vi "Capture_Python_Error.vi"(8 "error in (no error)":errorcluster, 11 "Error Message (start with ERROR)":string) -> (0 "error out":errorcluster)   [LabVIEW 2023]
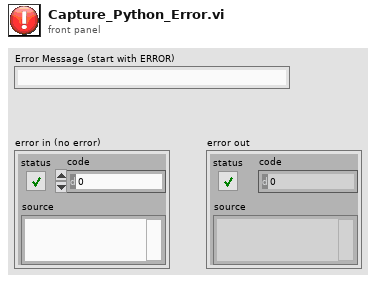
[diagram p1: front panel]
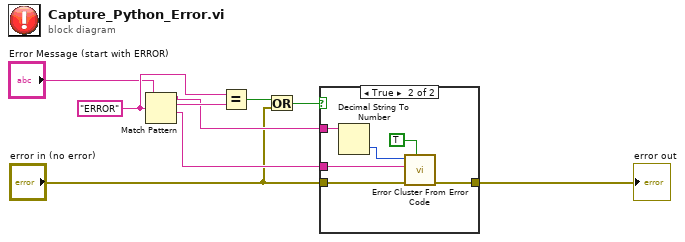
[diagram p0: block diagram]
diagram:
  w9 = "ERROR" ("regular expression")
  n1 = Match Pattern(string="Error Message (start with ERROR)", regular expression=w9) -> (before substring=w4:string, match substring=w8:string, after substring=w5:string)  [unwired: 1 in, 1 out]
  n2 = Equal?(x=w9, y=w8) -> (x = y?=w2:bool)
  n3 = Or(x=w2, y="error in (no error)") -> (x .or. y?=w1:bool)
  n4 = case shown="True" w1 {
    tunnel: "error in (no error)" -> [w10 w16]
    tunnel: [w10 w15] -> w6
    tunnel: w5 -> [_ w13]
    tunnel: w4 -> [_ w12]
    frame False {
    }
    frame True {
      n5 = Decimal String To Number(string=w12) -> (number=w11:i32)  [unwired: 2 in, 1 out]
      n6 = call <vilib>:"Error Cluster From Error Code.vi"("show call chain? (False)"=TRUE, "error in (no error)"=w16, "error message (\"\")"=w13, "error code (0)"=w11) -> ("error out"=w15:errorcluster)  [unwired: 5 in]
    }
  }
  "error out" <- w6
